vi "Flatten to CSV Record.vi"(7 "delimiter (,)":string=",", 10 "error in (no error)":errorcluster, 11 "row of strings":string[](array[string])) -> (2 "error out":errorcluster, 3 "CSV record":string)   [LabVIEW 2013, in "Robust CSV.lvlib"]
doc: "Convert 1D array of ANSI strings into a single CSV record (row).\n\nThe output CSV record string is formatted in accordance with RFC-4180 (see <b>http://tools.ietf.org/html/rfc4180<\\b>). \n\nAll cells containing double quotes (0x22), CR (0x0D) , LF (0x0A) or the delimiter character will be enclosed in double quotes. All double quote characters within a cell will be escaped using a second double quote character. The record ends with a CRLF.\n\nRev. 0.0 2014-02-20 Ryan Porter\n- First Draft\n\nRev 0.1 2014-10-30 Ryan Porter\n- Convert all CRLF and CR within a cell to LF\n- Changed end of record to CRLF for compatibility with Excel CSV import/export"
uses:
  Robust CSV.lvlib
panel:
  # "Flatten to CSV Record.vi\n\nConvert 1D array of ANSI strings into a single CSV record (row). The output CSV record string is formatted in accordance with RFC-4180 (see http://tools.ietf.org/html/rfc4180). \n\nAll cells containing double quotes (0x22), CR (0x0D) , LF (0x0A) or the delimiter character will be enclosed in double quotes. All double quote characters within a cell will be escaped using a second double quote character. A CRLF is appended to the end of the record."
  # "License: BSD (2-Clause) - http://opensource.org/licenses/BSD-2-Clause \n\nCopyright (c) 2014, Ryan Porter\nAll rights reserved."
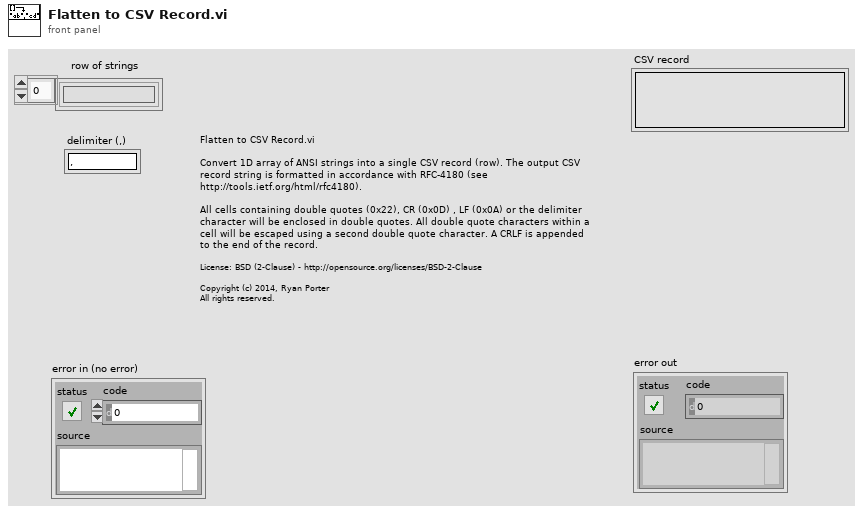
[diagram p1: front panel]
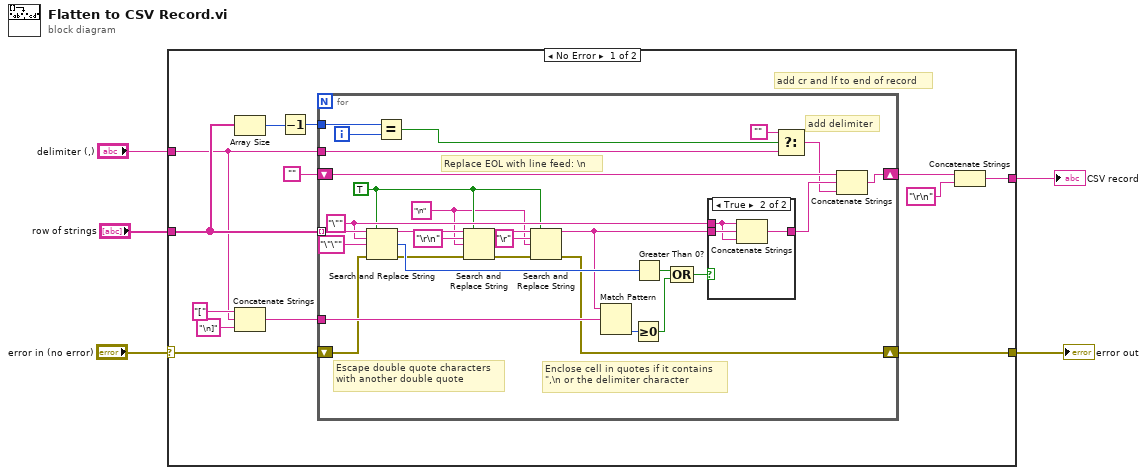
[diagram p0: block diagram]
diagram:
  n1 = case shown="No Error" "error in (no error)" {
    selector: "error in (no error)" -> [w7 w52]
    tunnel: "row of strings" -> [w16 _]
    tunnel: "delimiter (,)" -> [w13 _]
    tunnel: [w8 _] -> w3
    tunnel: [w6 w52] -> w1
    frame No Error {
      # "add cr and lf to end of record"
      n2 = Array Size(array=w16) -> (size(s)=w15:i32)
      n3 = Concatenate Strings("[", w13, "\n]") -> (w11:string)
      n4 = Decrement(x=w15) -> (x-1=w17:i32)
      n5 = for {
        tunnel: w16 -> [w47] mode=indexing
        tunnel: w11 -> [w40]
        shift-right: [w44] -> w10
        shift-left: "" -> [w43]
        tunnel: w13 -> [w37]
        tunnel: w17 -> [w34]
        shift-right: [w21] -> w6
        shift-left: w7 -> [w30]
        i -> [w39]
        w24 = "\n" ("replace string (\"\")")
        w26 = TRUE ("replace all? (F)")
        w45 = "\"" ("search string")
        # "Replace EOL with line feed: \\n"
        # "Escape double quote characters\nwith another double quote"
        # "Enclose cell in quotes if it contains\n\",\\n or the delimiter character"
        # "add delimiter"
        n6 = Search and Replace String(replace all?=w26, input string=w47, search string=w45, replace string="\"\"" ("replace string (\"\")"), error in=w30) -> (result string=w29:string, number of replacements=w33:i32, error out=w23:errorcluster)  [unwired: 3 in, 1 out]
        n7 = Equal?(x=w34, y=w39) -> (x = y?=w38:bool)
        n8 = Search and Replace String(replace all?=w26, input string=w29, search string="\r\n", replace string=w24, error in=w23) -> (result string=w27:string, error out=w22:errorcluster)  [unwired: 3 in, 2 out]
        n9 = Search and Replace String(replace all?=w26, input string=w27, search string="\r", replace string=w24, error in=w22) -> (result string=w20:string, error out=w21:errorcluster)  [unwired: 3 in, 2 out]
        n10 = Match Pattern(string=w20, regular expression=w40) -> (offset past match=w41:i32)  [unwired: 1 in, 3 out]
        n11 = Greater Or Equal To 0?(x=w41) -> (x >= 0?=w32:bool)
        n12 = Greater Than 0?(x=w33) -> (x > 0?=w19:bool)
        n13 = Compound Arithmetic op=OR(w19, w32) -> (w31:bool)
        n14 = case shown="True" w31 {
          tunnel: w20 -> [w48 w51]
          tunnel: w45 -> [_ w50]
          tunnel: [w48 w49] -> w42
          frame False {
          }
          frame True {
            n15 = Concatenate Strings(w50, w51, w50) -> (w49:string)
          }
        }
        n16 = Select(t="", s=w38, f=w37) -> (s? t:f=w35:string)
        n17 = Concatenate Strings(w43, w42, w35) -> (w44:string)
      }
      n18 = Concatenate Strings(w10, "\r\n") -> (w8:string)
    }
    frame Error {
    }
  }
  "CSV record" <- w3
  "error out" <- w1
